vi "Pre Launch Init.vi"(11 "Cooler in":refnum<class "Cooler.lvclass">=refnum) -> (0 "error out":errorcluster, 3 "Cooler out":refnum<class "Cooler.lvclass">)   [LabVIEW 2011]
doc: "Override this VI to do any initialization that you need to have happen during Launch. This VI is guaranteed to finish before Launch Actor.vi returns to its caller, whereas any initialization that you do in Actor Core.vi may not have finished running when the caller starts sending messages. This VI is invoked from within the actor, not the caller, which means that any refnums created in this VI will have the same lifetime as \"Actor Core.vi\". The actor object will already be populated with both its queue and its caller's queue, so the two protected accessor methods \"Get Queue For Sending To Caller.vi\" and \"Get Queue For Sending To Self.vi\" may be used if necessary."
uses:
  Dual Fan/Dual Fan.lvclass
  Water Level/Water Level.lvclass
  Cooler Service Alert Msg/Cooler Service Alert Msg.lvclass
  <vilib>/ActorFramework/Actor/Actor.lvclass
  Cooler.lvclass
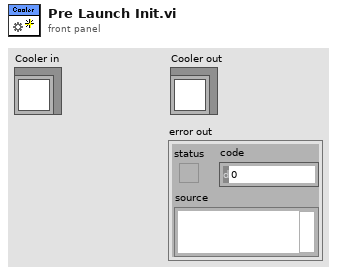
[diagram p1: front panel]
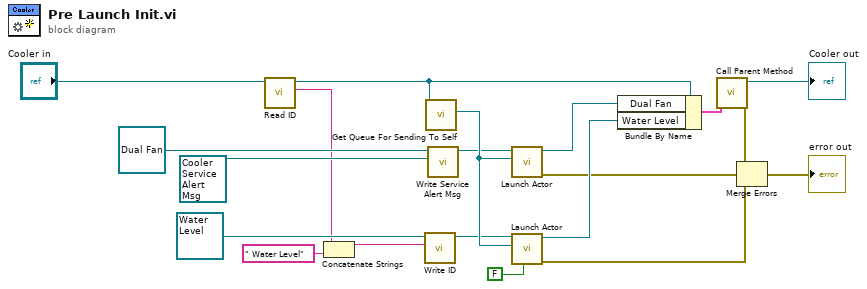
[diagram p0: block diagram]
diagram:
  n1 = call "Read ID.vi"("Level Controller in"="Cooler in") -> ("ID"=w4:string, "Level Controller out"=w6:refnum<class "Cooler.lvclass">)  [unwired: 8 in, 1 out]
  n2 = Concatenate Strings(w4, " Water Level" ("string")) -> (w3:string)
  n3 = call "Write ID.vi"("ID"=w3, "Level Controller in"=refnum<class "Water Level.lvclass"> refnum ("Water Level.lvclass")) -> ("Level Controller out"=w8:refnum<class "Water Level.lvclass">)  [unwired: 8 in, 1 out]
  n4 = call <vilib>:"Get Queue For Sending To Self.vi"("Actor in"=w6) -> ("To-Self Queue"=w14:refnum<class "Send Queue.lvclass">)  [unwired: 10 in]
  n5 = call "Write Service Alert Msg.vi"("Service Alert Msg.lvclass"=refnum<class "Cooler Service Alert Msg.lvclass"> refnum ("Cooler Service Alert Msg.lvclass"), "Dual Fan in"=refnum<class "Dual Fan.lvclass"> refnum ("Dual Fan.lvclass")) -> ("Dual Fan out"=w1:refnum<class "Dual Fan.lvclass">)  [unwired: 8 in, 1 out]
  n6 = call <vilib>:"Launch Actor.vi"("Actor-to-Caller Queue"=w14, "Actor"=w1) -> ("error out"=w11:errorcluster, "Caller-To-Actor Queue"=w13:refnum<class "Send Queue.lvclass">)  [unwired: 8 in]
  n7 = call <vilib>:"Launch Actor.vi"("Open Actor Core front panel? (F)"=FALSE, "Actor-to-Caller Queue"=w14, "Actor"=w8) -> ("error out"=w10:errorcluster, "Caller-To-Actor Queue"=w16:refnum<class "Send Queue.lvclass">)  [unwired: 7 in]
  n8 = Bundle By Name(cluster=w6, "Dual Fan"=w13, "Water Level"=w16) -> (w15:cluster{})
  n9 = call-parent "Call Parent Method"("Actor in"=w15) -> ("error out"=w20:errorcluster, "Actor out"=→"Cooler out":refnum<class "Cooler.lvclass">)  [unwired: 9 in]
  n10 = Merge Errors(w20, w11, w10) -> (→"error out":errorcluster)
